vi "Async Start recording video from CamServer.vi"(1 "Quality":i32=750 min=0 max=1000, 2 "Camera":T1="Travcam") -> (0 "Error out":errorcluster)   [LabVIEW 2015]
doc: "Asynchronously starts recording video from the selected camera on the camera server. The user must subsequently run the \"Async Stop and get video....\" vi to end the recording and save the video file."
uses:
  Camera enum/Camera enum.ctl
panel:
  # "PN 21/08/15"
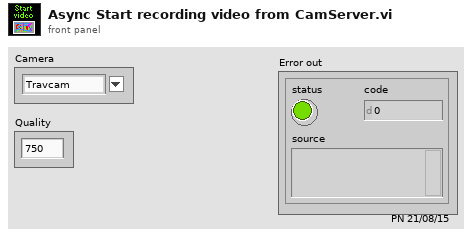
[diagram p1: front panel]
types:
  T1 = typedef "Camera enum.ctl" = string
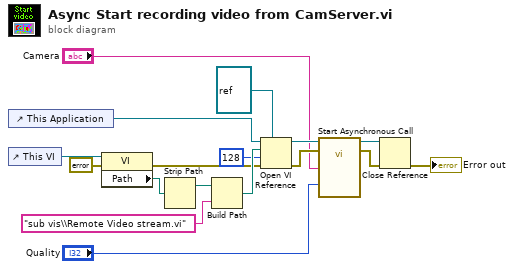
[diagram p0: block diagram]
diagram:
  n1 = control-ref of="This Application"() -> (w12:refnum<vi>)
  n2 = control-ref of="This VI"() -> (w17:refnum<vi>)
  n3 = property class="VI"(reference=w17, error in=errorcluster {"status"=FALSE, "code"=0, "source"=""} ("error in (no error)")) -> (error out=w14:errorcluster, "Path"=w10:path)  [unwired: 1 out]
  n4 = Strip Path(path=w10) -> (stripped path=w9:path)  [unwired: 1 out]
  n5 = Build Path(base path=w9, name or relative path="sub vis\\Remote Video stream.vi") -> (appended path=w15:path)
  n6 = Open VI Reference(type specifier VI Refnum (for type only)=refnum<vi> refnum, application reference (local)=w12, vi path=w15, options=128, error in (no error)=w14) -> (vi reference=w8:refnum<vi>, error out=w7:errorcluster)  [unwired: 1 in]
  n7 = call-by-ref "Start Asynchronous Call"(reference=w8, error in=w7, "Quality"="Quality", "Camera"="Camera") -> (reference out=w4:refnum<vi>, error out=w3:errorcluster)  [unwired: 1 out]
  n8 = Close Reference(reference=w4, error in (no error)=w3) -> (error out=→"Error out":errorcluster)
